vi "Read Power.vi"(11 "Harmonics in":refnum<class "Harmonics.lvclass">) -> (2 "Power":cluster{"List":dbl[], "Index":i32, "Last":bool}, 3 "Harmonics out":refnum<class "Harmonics.lvclass">)   [LabVIEW 2020, in "Harmonics.lvclass"]
uses:
  Harmonics.lvclass
  Harmonics.lvclass/Harmonics.ctl
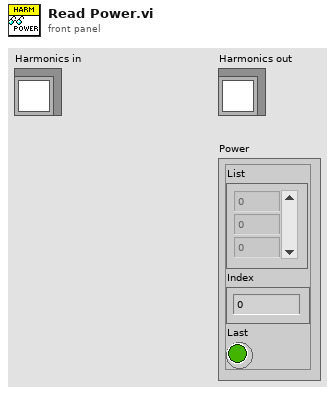
[diagram p1: front panel]
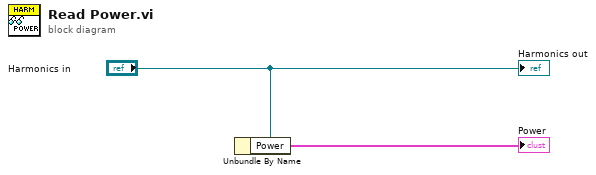
[diagram p0: block diagram]
diagram:
  n1 = Unbundle By Name("Harmonics in") -> ("Power"=→"Power":cluster{"List":dbl[], "Index":i32, "Last":bool})
  "Harmonics out" <- "Harmonics in"
